vi "Get Shared Variable Info - General - Refnum - Ver 2.vi"(8 "Error In":errorcluster, 9 "Type code":i32, 10 "Variable Refnum":variant) -> (0 "Error Out":errorcluster, 2 "Variable Name":string)   [LabVIEW 2014]
doc: "<B>Copyright</B>: (c) MHWirth 2015. All rights are reserved.\n\nThis SubVI reads the shared variable and returns it as a variant. It returns the size of the variable in two formats: numeric and string.\n\nSupported shared variable types:\nCode 1. Boolean\nCode 2 to 5. Int8/16/32/64\nCode 6 to 9. UInt8/16/32/64\nCode 10. Double\nCode 11. Single-precision\nCode 12. String\nCode 13-23 - 1D array of above types except string\n\n<B>Error 7001</B>: Unknown Data Type - Type Code Array (Int32) contains -1 indicating an unknown data type."
uses:
  Variable Refnum Cluster.ctl
  <resource>/objmgr/ni.var.rc
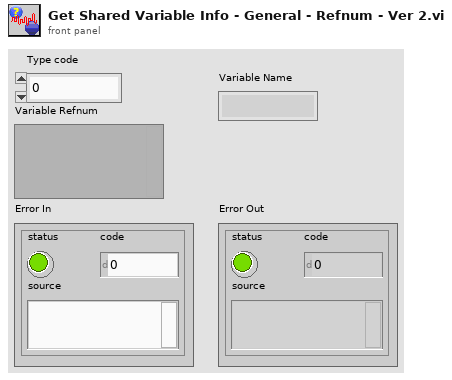
[diagram p1: front panel]
types:
  T1 = typedef "Variable Refnum Cluster.ctl" = cluster{"1":refnum<k21>, "2":refnum<k21>, "3":refnum<k21>, "4":refnum<k21>, "5":refnum<k21>, "6":refnum<k21>, "7":refnum<k21>, "8":refnum<k21>, "9":refnum<k21>, "10":refnum<k21>, "11":refnum<k21>, "12":refnum<k21>, "13":refnum<k21>, "14":refnum<k21>, "15":refnum<k21>, "16":refnum<k21>, "17":refnum<k21>, "18":refnum<k21>, "19":refnum<k21>, "20":refnum<k21>, "21":refnum<k21>, "22":refnum<k21>, "23":refnum<k21>, "24":refnum<k21>, "25":refnum<k21>, "26":refnum<k21>, "27":refnum<k21>, "28":refnum<k21>, "29":refnum<k21>, "30":refnum<k21>, "31":refnum<k21>, "32":refnum<k21>, "33":refnum<k21>, "34":refnum<k21>, "35":refnum<k21>, "36":refnum<k21>}
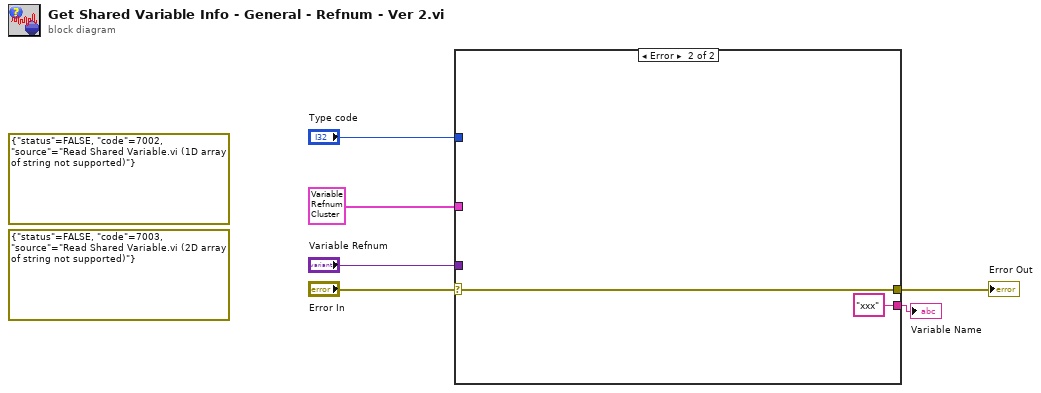
[diagram p0: block diagram]
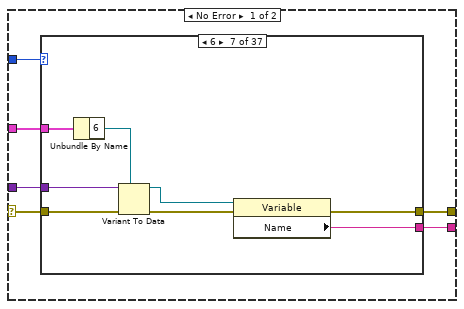
[diagram p2: hidden frame]
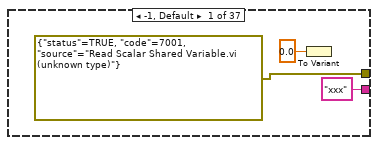
[diagram p3: hidden frame]
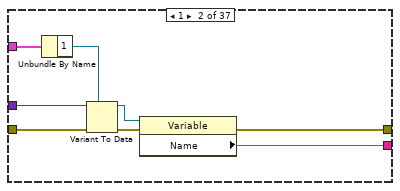
[diagram p4: hidden frame]
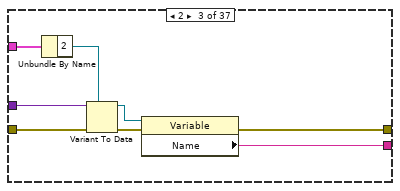
[diagram p5: hidden frame]
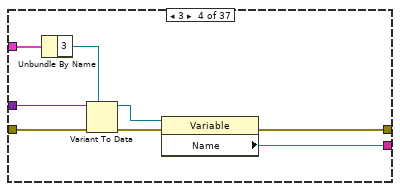
[diagram p6: hidden frame]
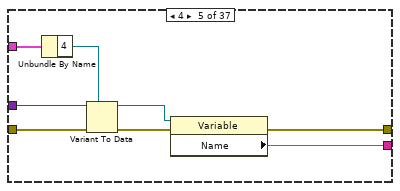
[diagram p7: hidden frame]
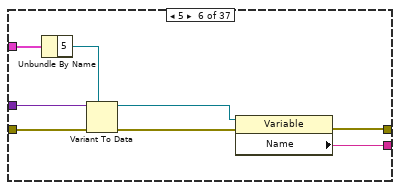
[diagram p8: hidden frame]
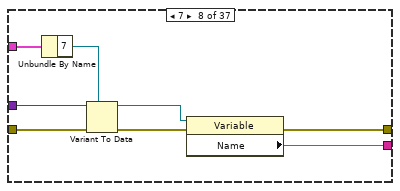
[diagram p9: hidden frame]
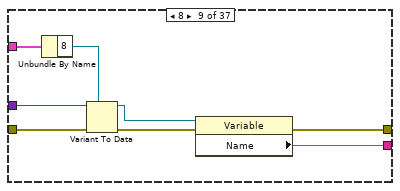
[diagram p10: hidden frame]
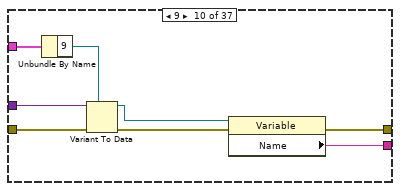
[diagram p11: hidden frame]
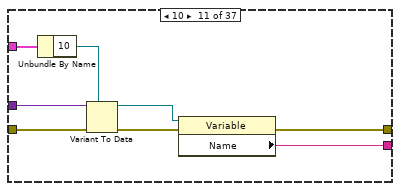
[diagram p12: hidden frame]
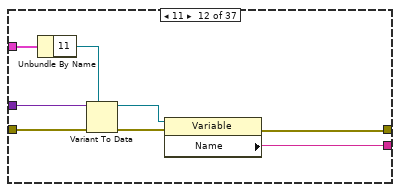
[diagram p13: hidden frame]
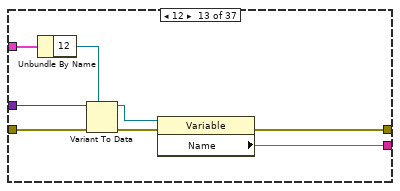
[diagram p14: hidden frame]
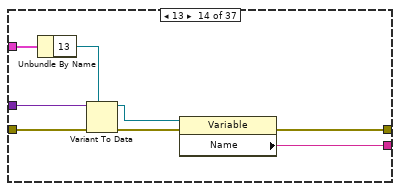
[diagram p15: hidden frame]
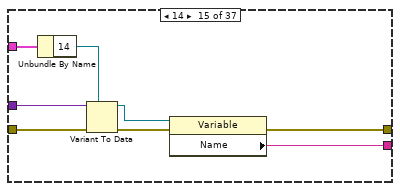
[diagram p16: hidden frame]
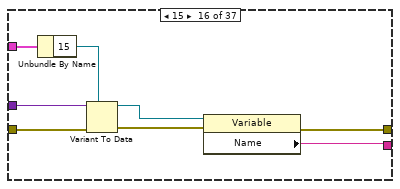
[diagram p17: hidden frame]
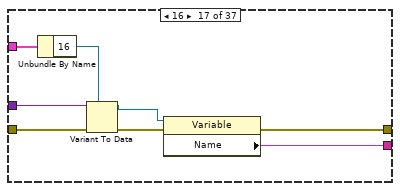
[diagram p18: hidden frame]
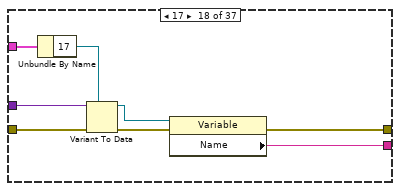
[diagram p19: hidden frame]
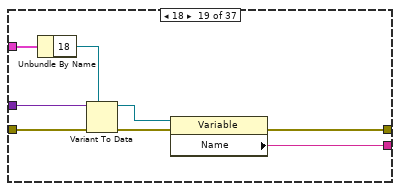
[diagram p20: hidden frame]
diagram:
  (unwired) errorcluster {"status"=FALSE, "code"=7002, "source"="Read Shared Variable.vi (1D array of string not supported)"} ("Error In")
  (unwired) errorcluster {"status"=FALSE, "code"=7003, "source"="Read Shared Variable.vi (2D array of string not supported)"} ("Error In")
  n1 = case shown="Error" "Error In" {
    selector: "Error In" -> [w9 w305]
    tunnel: "Type code" -> [w12 _]
    tunnel: "Variable Refnum" -> [w11 _]
    tunnel: T1 {"1"="", "2"="", "3"="", "4"="", "5"="", "6"="", "7"="", "8"="", "9"="", "10"="", "11"="", "12"="", "13"="", "14"="", "15"="", "16"="", "17"="", "18"="", "19"="", "20"="", "21"="", "22"="", "23"="", "24"="", "25"="", "26"="", "27"="", "28"="", "29"="", "30"="", "31"="", "32"="", "33"="", "34"="", "35"="", "36"=""} ("output cluster") -> [w10 _]
    tunnel: [w8 w305] -> w2
    tunnel: [w7 "xxx" ("Name")] -> w1
    frame No Error {
      n2 = case shown="6" w12 {
        tunnel: w11 -> [_ w23 w31 w39 w47 w55 w63 w71 w79 w87 w95 w103 w111 w119 w127 w135 w143 w151 w159 w167 w175 w183 w191 w199 w207 w215 w223 w231 w239 w247 w255 w263 w271 w279 w287 w295 w303]
        tunnel: w10 -> [_ w22 w30 w38 w46 w54 w62 w70 w78 w86 w94 w102 w110 w118 w126 w134 w142 w150 w158 w166 w174 w182 w190 w198 w206 w214 w222 w230 w238 w246 w254 w262 w270 w278 w286 w294 w302]
        tunnel: w9 -> [_ w20 w28 w36 w44 w52 w60 w68 w76 w84 w92 w100 w108 w116 w124 w132 w140 w148 w156 w164 w172 w180 w188 w196 w204 w212 w220 w228 w236 w244 w252 w260 w268 w276 w284 w292 w300]
        tunnel: [errorcluster {"status"=TRUE, "code"=7001, "source"="Read Scalar Shared Variable.vi (unknown type)"} ("error constant") w17 w25 w33 w41 w49 w57 w65 w73 w81 w89 w97 w105 w112 w121 w131 w138 w145 w154 w162 w171 w178 w185 w193 w201 w210 w219 w227 w234 w243 w250 w257 w266 w273 w282 w291 w299] -> w8
        tunnel: ["xxx" ("Name") w16 w24 w32 w40 w48 w56 w64 w72 w80 w88 w96 w104 w113 w120 w128 w137 w144 w153 w160 w170 w177 w184 w192 w200 w209 w218 w225 w232 w242 w249 w256 w265 w272 w283 w290 w296] -> w7
        frame -1, Default {
          n3 = To Variant(anything=0.0) -> ()  [unwired: 1 out]
        }
        frame 1 {
          n4 = Unbundle By Name(w22) -> ("1"=w21:refnum<k21>)
          n5 = Variant To Data(error in=w20, type=w21, Variant=w23) -> (data=w19:refnum<k21>, error out=w18:errorcluster)
          n6 = property class="Variable"(reference=w19, error in=w18) -> (error out=w17:errorcluster, "Name"=w16:string)  [unwired: 1 out]
        }
        frame 2 {
          n7 = Unbundle By Name(w30) -> ("2"=w29:refnum<k21>)
          n8 = Variant To Data(error in=w28, type=w29, Variant=w31) -> (data=w26:refnum<k21>, error out=w27:errorcluster)
          n9 = property class="Variable"(reference=w26, error in=w27) -> (error out=w25:errorcluster, "Name"=w24:string)  [unwired: 1 out]
        }
        frame 3 {
          n10 = Unbundle By Name(w38) -> ("3"=w37:refnum<k21>)
          n11 = Variant To Data(error in=w36, type=w37, Variant=w39) -> (data=w34:refnum<k21>, error out=w35:errorcluster)
          n12 = property class="Variable"(reference=w34, error in=w35) -> (error out=w33:errorcluster, "Name"=w32:string)  [unwired: 1 out]
        }
        frame 4 {
          n13 = Unbundle By Name(w46) -> ("4"=w45:refnum<k21>)
          n14 = Variant To Data(error in=w44, type=w45, Variant=w47) -> (data=w42:refnum<k21>, error out=w43:errorcluster)
          n15 = property class="Variable"(reference=w42, error in=w43) -> (error out=w41:errorcluster, "Name"=w40:string)  [unwired: 1 out]
        }
        frame 5 {
          n16 = Unbundle By Name(w54) -> ("5"=w53:refnum<k21>)
          n17 = Variant To Data(error in=w52, type=w53, Variant=w55) -> (data=w50:refnum<k21>, error out=w51:errorcluster)
          n18 = property class="Variable"(reference=w50, error in=w51) -> (error out=w49:errorcluster, "Name"=w48:string)  [unwired: 1 out]
        }
        frame 6 {
          n19 = Unbundle By Name(w62) -> ("6"=w61:refnum<k21>)
          n20 = Variant To Data(error in=w60, type=w61, Variant=w63) -> (data=w58:refnum<k21>, error out=w59:errorcluster)
          n21 = property class="Variable"(reference=w58, error in=w59) -> (error out=w57:errorcluster, "Name"=w56:string)  [unwired: 1 out]
        }
        frame 7 {
          n22 = Unbundle By Name(w70) -> ("7"=w69:refnum<k21>)
          n23 = Variant To Data(error in=w68, type=w69, Variant=w71) -> (data=w66:refnum<k21>, error out=w67:errorcluster)
          n24 = property class="Variable"(reference=w66, error in=w67) -> (error out=w65:errorcluster, "Name"=w64:string)  [unwired: 1 out]
        }
        frame 8 {
          n25 = Unbundle By Name(w78) -> ("8"=w77:refnum<k21>)
          n26 = Variant To Data(error in=w76, type=w77, Variant=w79) -> (data=w74:refnum<k21>, error out=w75:errorcluster)
          n27 = property class="Variable"(reference=w74, error in=w75) -> (error out=w73:errorcluster, "Name"=w72:string)  [unwired: 1 out]
        }
        frame 9 {
          n28 = Unbundle By Name(w86) -> ("9"=w85:refnum<k21>)
          n29 = Variant To Data(error in=w84, type=w85, Variant=w87) -> (data=w82:refnum<k21>, error out=w83:errorcluster)
          n30 = property class="Variable"(reference=w82, error in=w83) -> (error out=w81:errorcluster, "Name"=w80:string)  [unwired: 1 out]
        }
        frame 10 {
          n31 = Unbundle By Name(w94) -> ("10"=w93:refnum<k21>)
          n32 = Variant To Data(error in=w92, type=w93, Variant=w95) -> (data=w90:refnum<k21>, error out=w91:errorcluster)
          n33 = property class="Variable"(reference=w90, error in=w91) -> (error out=w89:errorcluster, "Name"=w88:string)  [unwired: 1 out]
        }
        frame 11 {
          n34 = Unbundle By Name(w102) -> ("11"=w101:refnum<k21>)
          n35 = Variant To Data(error in=w100, type=w101, Variant=w103) -> (data=w98:refnum<k21>, error out=w99:errorcluster)
          n36 = property class="Variable"(reference=w98, error in=w99) -> (error out=w97:errorcluster, "Name"=w96:string)  [unwired: 1 out]
        }
        frame 12 {
          n37 = Unbundle By Name(w110) -> ("12"=w109:refnum<k21>)
          n38 = Variant To Data(error in=w108, type=w109, Variant=w111) -> (data=w107:refnum<k21>, error out=w106:errorcluster)
          n39 = property class="Variable"(reference=w107, error in=w106) -> (error out=w105:errorcluster, "Name"=w104:string)  [unwired: 1 out]
        }
        frame 13 {
          n40 = Unbundle By Name(w118) -> ("13"=w117:refnum<k21>)
          n41 = Variant To Data(error in=w116, type=w117, Variant=w119) -> (data=w114:refnum<k21>, error out=w115:errorcluster)
          n42 = property class="Variable"(reference=w114, error in=w115) -> (error out=w112:errorcluster, "Name"=w113:string)  [unwired: 1 out]
        }
        frame 14 {
          n43 = Unbundle By Name(w126) -> ("14"=w125:refnum<k21>)
          n44 = Variant To Data(error in=w124, type=w125, Variant=w127) -> (data=w122:refnum<k21>, error out=w123:errorcluster)
          n45 = property class="Variable"(reference=w122, error in=w123) -> (error out=w121:errorcluster, "Name"=w120:string)  [unwired: 1 out]
        }
        frame 15 {
          n46 = Unbundle By Name(w134) -> ("15"=w133:refnum<k21>)
          n47 = Variant To Data(error in=w132, type=w133, Variant=w135) -> (data=w129:refnum<k21>, error out=w130:errorcluster)
          n48 = property class="Variable"(reference=w129, error in=w130) -> (error out=w131:errorcluster, "Name"=w128:string)  [unwired: 1 out]
        }
        frame 16 {
          n49 = Unbundle By Name(w142) -> ("16"=w141:refnum<k21>)
          n50 = Variant To Data(error in=w140, type=w141, Variant=w143) -> (data=w136:refnum<k21>, error out=w139:errorcluster)
          n51 = property class="Variable"(reference=w136, error in=w139) -> (error out=w138:errorcluster, "Name"=w137:string)  [unwired: 1 out]
        }
        frame 17 {
          n52 = Unbundle By Name(w150) -> ("17"=w149:refnum<k21>)
          n53 = Variant To Data(error in=w148, type=w149, Variant=w151) -> (data=w146:refnum<k21>, error out=w147:errorcluster)
          n54 = property class="Variable"(reference=w146, error in=w147) -> (error out=w145:errorcluster, "Name"=w144:string)  [unwired: 1 out]
        }
        frame 18 {
          n55 = Unbundle By Name(w158) -> ("18"=w157:refnum<k21>)
          n56 = Variant To Data(error in=w156, type=w157, Variant=w159) -> (data=w152:refnum<k21>, error out=w155:errorcluster)
          n57 = property class="Variable"(reference=w152, error in=w155) -> (error out=w154:errorcluster, "Name"=w153:string)  [unwired: 1 out]
        }
        frame 19 {
          n58 = Unbundle By Name(w166) -> ("19"=w165:refnum<k21>)
          n59 = Variant To Data(error in=w164, type=w165, Variant=w167) -> (data=w161:refnum<k21>, error out=w163:errorcluster)
          n60 = property class="Variable"(reference=w161, error in=w163) -> (error out=w162:errorcluster, "Name"=w160:string)  [unwired: 1 out]
        }
        frame 20 {
          n61 = Unbundle By Name(w174) -> ("20"=w173:refnum<k21>)
          n62 = Variant To Data(error in=w172, type=w173, Variant=w175) -> (data=w168:refnum<k21>, error out=w169:errorcluster)
          n63 = property class="Variable"(reference=w168, error in=w169) -> (error out=w171:errorcluster, "Name"=w170:string)  [unwired: 1 out]
        }
        frame 21 {
          n64 = Unbundle By Name(w182) -> ("21"=w181:refnum<k21>)
          n65 = Variant To Data(error in=w180, type=w181, Variant=w183) -> (data=w176:refnum<k21>, error out=w179:errorcluster)
          n66 = property class="Variable"(reference=w176, error in=w179) -> (error out=w178:errorcluster, "Name"=w177:string)  [unwired: 1 out]
        }
        frame 22 {
          n67 = Unbundle By Name(w190) -> ("22"=w189:refnum<k21>)
          n68 = Variant To Data(error in=w188, type=w189, Variant=w191) -> (data=w186:refnum<k21>, error out=w187:errorcluster)
          n69 = property class="Variable"(reference=w186, error in=w187) -> (error out=w185:errorcluster, "Name"=w184:string)  [unwired: 1 out]
        }
        frame 23 {
          n70 = Unbundle By Name(w198) -> ("23"=w197:refnum<k21>)
          n71 = Variant To Data(error in=w196, type=w197, Variant=w199) -> (data=w194:refnum<k21>, error out=w195:errorcluster)
          n72 = property class="Variable"(reference=w194, error in=w195) -> (error out=w193:errorcluster, "Name"=w192:string)  [unwired: 1 out]
        }
        frame 24 {
          n73 = Unbundle By Name(w206) -> ("24"=w205:refnum<k21>)
          n74 = Variant To Data(error in=w204, type=w205, Variant=w207) -> (data=w202:refnum<k21>, error out=w203:errorcluster)
          n75 = property class="Variable"(reference=w202, error in=w203) -> (error out=w201:errorcluster, "Name"=w200:string)  [unwired: 1 out]
        }
        frame 25 {
          n76 = Unbundle By Name(w214) -> ("25"=w213:refnum<k21>)
          n77 = Variant To Data(error in=w212, type=w213, Variant=w215) -> (data=w208:refnum<k21>, error out=w211:errorcluster)
          n78 = property class="Variable"(reference=w208, error in=w211) -> (error out=w210:errorcluster, "Name"=w209:string)  [unwired: 1 out]
        }
        frame 26 {
          n79 = Unbundle By Name(w222) -> ("26"=w221:refnum<k21>)
          n80 = Variant To Data(error in=w220, type=w221, Variant=w223) -> (data=w216:refnum<k21>, error out=w217:errorcluster)
          n81 = property class="Variable"(reference=w216, error in=w217) -> (error out=w219:errorcluster, "Name"=w218:string)  [unwired: 1 out]
        }
        frame 27 {
          n82 = Unbundle By Name(w230) -> ("27"=w229:refnum<k21>)
          n83 = Variant To Data(error in=w228, type=w229, Variant=w231) -> (data=w224:refnum<k21>, error out=w226:errorcluster)
          n84 = property class="Variable"(reference=w224, error in=w226) -> (error out=w227:errorcluster, "Name"=w225:string)  [unwired: 1 out]
        }
        frame 28 {
          n85 = Unbundle By Name(w238) -> ("28"=w237:refnum<k21>)
          n86 = Variant To Data(error in=w236, type=w237, Variant=w239) -> (data=w233:refnum<k21>, error out=w235:errorcluster)
          n87 = property class="Variable"(reference=w233, error in=w235) -> (error out=w234:errorcluster, "Name"=w232:string)  [unwired: 1 out]
        }
        frame 29 {
          n88 = Unbundle By Name(w246) -> ("29"=w245:refnum<k21>)
          n89 = Variant To Data(error in=w244, type=w245, Variant=w247) -> (data=w240:refnum<k21>, error out=w241:errorcluster)
          n90 = property class="Variable"(reference=w240, error in=w241) -> (error out=w243:errorcluster, "Name"=w242:string)  [unwired: 1 out]
        }
        frame 30 {
          n91 = Unbundle By Name(w254) -> ("30"=w253:refnum<k21>)
          n92 = Variant To Data(error in=w252, type=w253, Variant=w255) -> (data=w248:refnum<k21>, error out=w251:errorcluster)
          n93 = property class="Variable"(reference=w248, error in=w251) -> (error out=w250:errorcluster, "Name"=w249:string)  [unwired: 1 out]
        }
        frame 31 {
          n94 = Unbundle By Name(w262) -> ("31"=w261:refnum<k21>)
          n95 = Variant To Data(error in=w260, type=w261, Variant=w263) -> (data=w258:refnum<k21>, error out=w259:errorcluster)
          n96 = property class="Variable"(reference=w258, error in=w259) -> (error out=w257:errorcluster, "Name"=w256:string)  [unwired: 1 out]
        }
        frame 32 {
          n97 = Unbundle By Name(w270) -> ("32"=w269:refnum<k21>)
          n98 = Variant To Data(error in=w268, type=w269, Variant=w271) -> (data=w264:refnum<k21>, error out=w267:errorcluster)
          n99 = property class="Variable"(reference=w264, error in=w267) -> (error out=w266:errorcluster, "Name"=w265:string)  [unwired: 1 out]
        }
        frame 33 {
          n100 = Unbundle By Name(w278) -> ("33"=w277:refnum<k21>)
          n101 = Variant To Data(error in=w276, type=w277, Variant=w279) -> (data=w274:refnum<k21>, error out=w275:errorcluster)
          n102 = property class="Variable"(reference=w274, error in=w275) -> (error out=w273:errorcluster, "Name"=w272:string)  [unwired: 1 out]
        }
        frame 34 {
          n103 = Unbundle By Name(w286) -> ("34"=w285:refnum<k21>)
          n104 = Variant To Data(error in=w284, type=w285, Variant=w287) -> (data=w280:refnum<k21>, error out=w281:errorcluster)
          n105 = property class="Variable"(reference=w280, error in=w281) -> (error out=w282:errorcluster, "Name"=w283:string)  [unwired: 1 out]
        }
        frame 35 {
          n106 = Unbundle By Name(w294) -> ("35"=w293:refnum<k21>)
          n107 = Variant To Data(error in=w292, type=w293, Variant=w295) -> (data=w288:refnum<k21>, error out=w289:errorcluster)
          n108 = property class="Variable"(reference=w288, error in=w289) -> (error out=w291:errorcluster, "Name"=w290:string)  [unwired: 1 out]
        }
        frame 36 {
          n109 = Unbundle By Name(w302) -> ("36"=w301:refnum<k21>)
          n110 = Variant To Data(error in=w300, type=w301, Variant=w303) -> (data=w297:refnum<k21>, error out=w298:errorcluster)
          n111 = property class="Variable"(reference=w297, error in=w298) -> (error out=w299:errorcluster, "Name"=w296:string)  [unwired: 1 out]
        }
      }
    }
    frame Error {
    }
  }
  "Error Out" <- w2
  "Variable Name" <- w1
